vi "Robotiq Control.vi"() -> ()   [LabVIEW 2011]
uses:
  Classes/MF3/MF3.lvclass
panel:
  out "motor currents":dbl[](array[numeric])
  out "Finger Positions":T1
  out "error out":errorcluster
  in  "Motors PI Gains":T2
  in  "Stop":bool
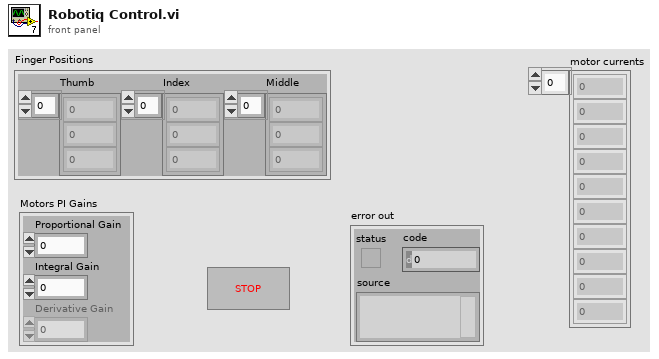
[diagram p1: front panel]
types:
  T1 = cluster{"Thumb":dbl[], "Index":dbl[], "Middle":dbl[]}
  T2 = cluster{"Proportional Gain":i16, "Integral Gain":i16, "Derivative Gain":i16}
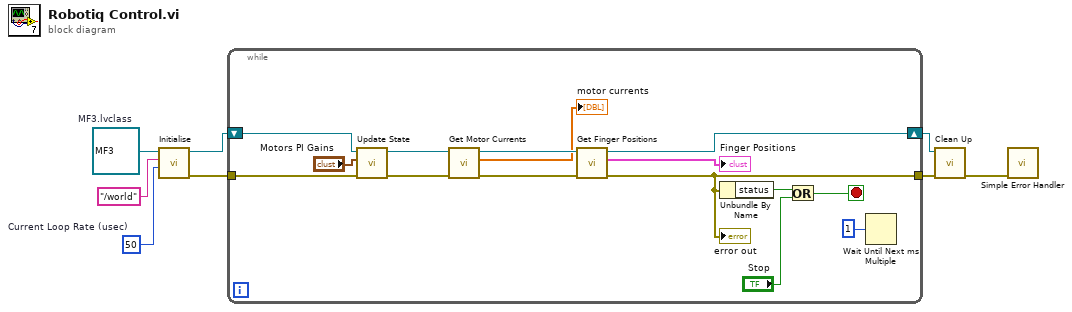
[diagram p0: block diagram]
diagram:
  w6 = u32 50  # Current Loop Rate (usec)
  w8 = refnum<class "MF3.lvclass"> refnum  # MF3.lvclass
  n1 = call "Initialise.vi"("Current Loop Rate (usec)"=w6, "frame"="/world", "MF3 in"=w8) -> ("error out"=w4:errorcluster, "MF3 out"=w5:refnum<class "MF3.lvclass">)  [unwired: 7 in]
  n2 = while {
    shift-right: [w16] -> w2
    shift-left: w5 -> [w19]
    tunnel: w4 -> [w18]
    tunnel: [w17] -> w3
    stop <- w23 stop-if-true
    n3 = call "Update State.vi"("error in (no error)"=w18, "Motors Gains"="Motors PI Gains", "MF3 in"=w19) -> ("error out"=w12:errorcluster, "MF3 out"=w13:refnum<class "MF3.lvclass">)  [unwired: 6 in, 1 out]
    n4 = call "Get Motor Currents.vi"("error in (no error)"=w12, "MF3 in"=w13) -> ("error out"=w10:errorcluster, "motor currents"=→"motor currents":dbl[], "MF3 out"=w11:refnum<class "MF3.lvclass">)  [unwired: 7 in]
    n5 = call "Get Finger Positions.vi"("error in (no error)"=w10, "MF3 in"=w11) -> ("error out"=w17:errorcluster, "Finger Positions"=→"Finger Positions":T1, "MF3 out"=w16:refnum<class "MF3.lvclass">)  [unwired: 7 in]
    "error out" <- w17
    n6 = Unbundle By Name(w17) -> ("status"=w21:bool)
    n7 = Or(x=w21, y="Stop") -> (x .or. y?=w23:bool)
    n8 = Wait Until Next ms Multiple(millisecond multiple=u32 1) -> ()  [unwired: 1 out]
  }
  n9 = call "Clean Up.vi"("error in (no error)"=w3, "MF3 in"=w2) -> ("error out"=w1:errorcluster)  [unwired: 8 in, 1 out]
  n10 = call <vilib>:"Simple Error Handler.vi"("error in (no error)"=w1) -> ()  [unwired: 4 in, 5 out]
